vi "armTrigger.vi"(8 "error in (no error)":errorcluster, 10 "Trigger default: board0 (t = 0)":T1, 11 "Refnum in":refnum<k20>) -> (0 "error out":errorcluster, 2 "IRQ":i32, 3 "Refnum out":refnum<k20>)   [LabVIEW 2014]
uses:
  TriggerChannel.ctl
  <vilib>/Utility/error.llb/Error Cluster From Error Code.vi
  <vilib>/rvi/interface/nirviMethod/nirviMethod.xnode
  FPGA Bitfiles/W7XBolo2017_FPGATarget_fmain2014_9xlV3GyHFfo.lvbitx
  f_main_2014.vi
  <vilib>/FPGAPlugInAG/PCI-7813R/niLvFpga_AcknowledgeIrq_PCI-7813R.vi
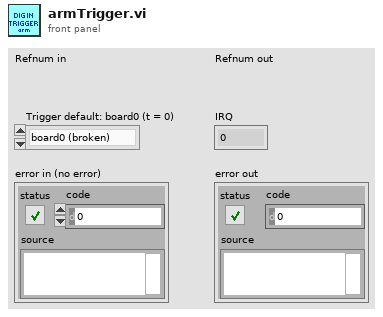
[diagram p1: front panel]
types:
  T1 = typedef "TriggerChannel.ctl" = enum16{"board0 (broken)", "board1 (t = -60sec)", "board2 (t = 0sec)"}
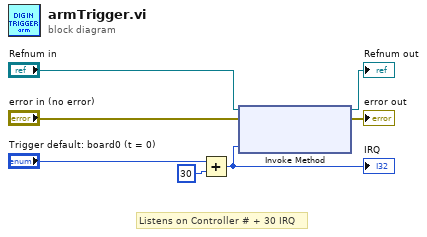
[diagram p0: block diagram]
diagram:
  # "Listens on Controller # + 30 IRQ"
  n1 = Add(x="Trigger default: board0 (t = 0)", y=30 ("IRQ Number(s)")) -> (x+y=w7:i32)
  "IRQ" <- w7
  n2 = xnode "Invoke Method"("FPGA VI Reference In"="Refnum in", "error in"="error in (no error)", "IRQ Number(s)"=w7) -> ("FPGA VI Reference Out"=→"Refnum out":refnum<k20>, "error out"=→"error out":errorcluster)
